vi "Enter Number.vi"(8 "error in":errorcluster, 10 "Numeric Control":dbl, 11 "Message":string) -> (0 "error out":errorcluster, 2 "Numeric Value":dbl)   [LabVIEW 2017]
panel:
  in  "OK Button":bool
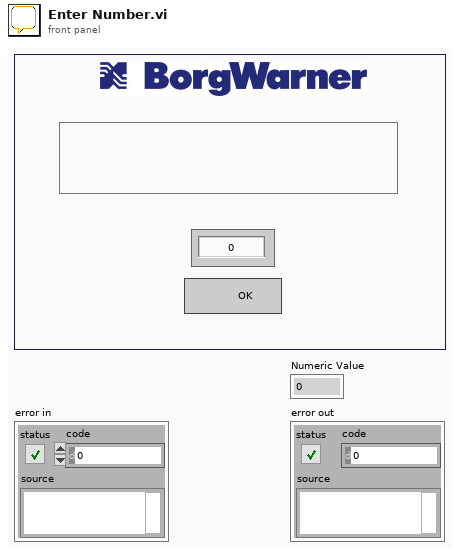
[diagram p1: front panel]
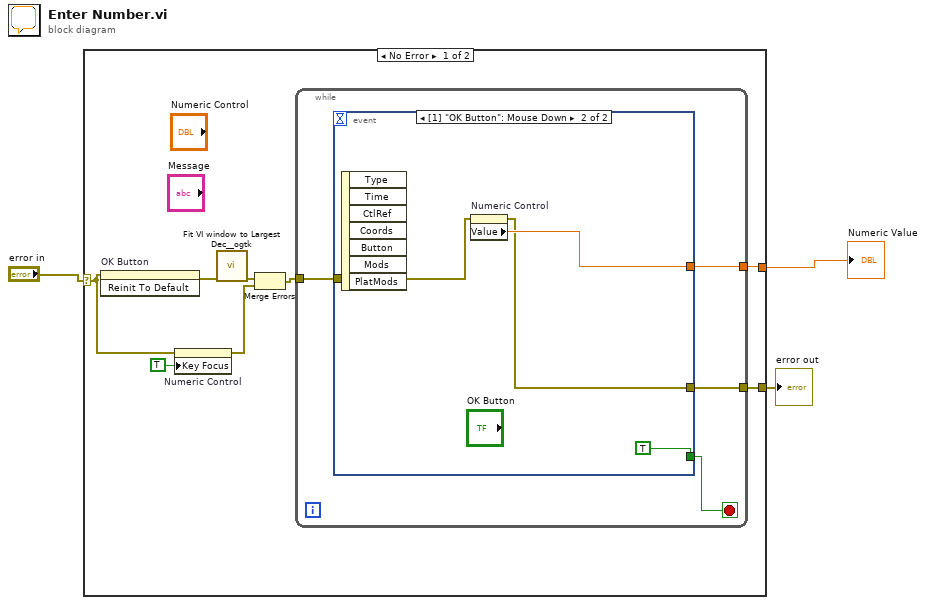
[diagram p0: block diagram]
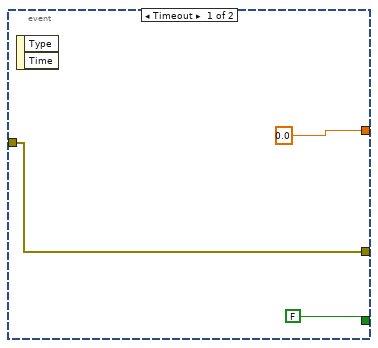
[diagram p2: hidden frame]
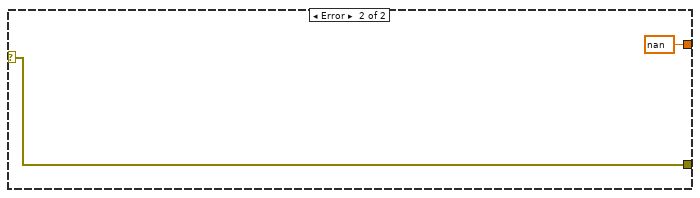
[diagram p3: hidden frame]
diagram:
  n1 = case shown="No Error" "error in" {
    selector: "error in" -> [w7 w23]
    tunnel: [w10 nan ("Numeric Control")] -> w3
    tunnel: [w9 w23] -> w1
    frame No Error {
      n2 = invoke on="OK Button" class="Bool" method="Reinit To Default"(error in=w7) -> (error out=w11:errorcluster)  [unwired: 2 in, 2 out]
      n3 = property on="Numeric Control" class="DigNum (strict)"(error in=w7, "Key Focus"=TRUE) -> (error out=w5:errorcluster)  [unwired: 1 in, 1 out]
      n4 = call <userlib>:"Fit VI window to Largest Dec__ogtk.vi"("error in (no error)"=w11) -> ("error out"=w6:errorcluster)  [unwired: 5 in, 1 out]
      n5 = Merge Errors(w6, w5) -> (w4:errorcluster)
      n6 = while {
        tunnel: w4 -> [w15]
        tunnel: [w14] -> w10
        tunnel: [w13] -> w9
        stop <- w12 stop-if-true
        n7 = event shown="[1] \"OK Button\": Mouse Down" {
          selector: _ -> [_ _]
          dyn-events: _ -> [_ _]
          timeout: _ -> [_ _]
          tunnel: w15 -> [w18 w20]
          tunnel: [0.0 ("Numeric Control") w21] -> w14
          tunnel: [w18 w19] -> w13
          tunnel: [FALSE TRUE] -> w12
          event Timeout {
            n8 = event-data() -> ()  [unwired: 1 in, 2 out]
          }
          event "OK Button": Mouse Down {
            n9 = event-data() -> ()  [unwired: 1 in, 7 out]
            n10 = property on="Numeric Control" class="DigNum (strict)"(error in=w20) -> (error out=w19:errorcluster, "Value"=w21:dbl)  [unwired: 1 in, 1 out]
          }
        }
      }
    }
    frame Error {
    }
  }
  "Numeric Value" <- w3
  "error out" <- w1
